vi "LVH5Rget_obj_type (DSet).vi"(6 "error in (no error)":errorcluster, 8 "HDF5 Object Reference":T2, 9 "HDF5 Location Ref":T3) -> (0 "error out":errorcluster, 2 "Object Type":T1 items=["H5O_TYPE_GROUP", "H5O_TYPE_DATASET", "H5O_NAMED_DATATYPE"], 3 "HDF5 Location Ref out":T3)   [LabVIEW 2017]
doc: "Retrieves the type of object that an object reference points to."
uses:
  <vilib>/UPVI/lvhdf5/library.llb/HDF5 Ref.ctl
  <vilib>/UPVI/lvhdf5/reference.llb/H5R Dataset Region Ref.ctl
  <vilib>/UPVI/lvhdf5/object.llb/H5O_type_t.ctl
  <vilib>/UPVI/lvhdf5/h5helper.dll
panel:
  # "LVHDF5 Toolkit\nCopyright (c) 2005-2013 by Jason D. Sommerville\nCopyright (c) 2014 by UPVI, LLC.\n\nThis use and distribution of this file is governed by the terms found in \nLICENSE.txt distributed with this toolkit and installed at\n <user.lib>\\_lvhdf5\\LICENSE.txt"
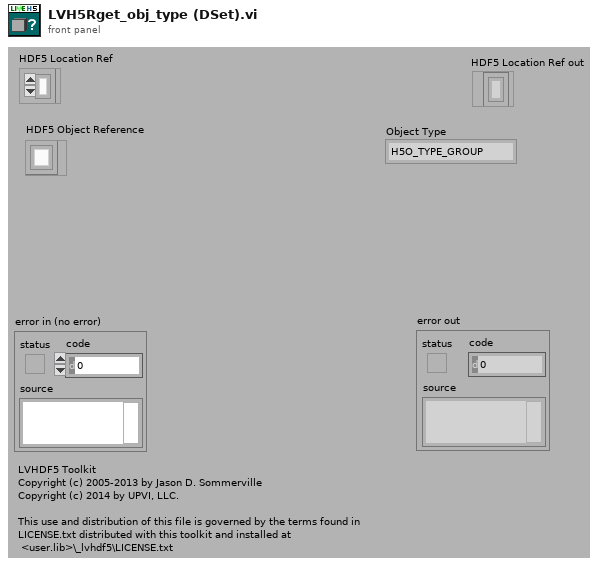
[diagram p1: front panel]
types:
  T1 = typedef "H5O_type_t.ctl" = i32
  T2 = typedef "H5R Dataset Region Ref.ctl" = refnum<k1>
  T3 = typedef "HDF5 Ref.ctl" = refnum<k1>
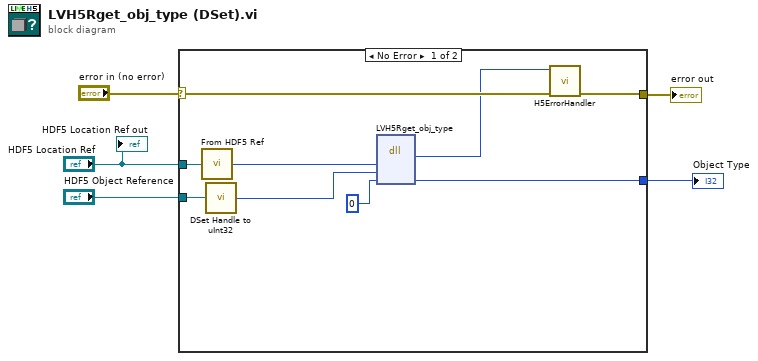
[diagram p0: block diagram]
diagram:
  n1 = case shown="No Error" "error in (no error)" {
    selector: "error in (no error)" -> [w14 w15]
    tunnel: [w13 w15] -> w4
    tunnel: "HDF5 Location Ref" -> [w12 _]
    tunnel: "HDF5 Object Reference" -> [w7 _]
    tunnel: [w8 _] -> w1
    frame No Error {
      n2 = call <vilib>:"From HDF5 Ref.vi"("HDF5 Ref"=w12) -> ("I32"=w11:i32)
      n3 = call <vilib>:"DSet Handle to uInt32.vi"("HDF5 Reference Type"=w7) -> ("Handle"=w6:u32)
      n4 = dll-call lib="C:/Program Files/National Instruments/LabVIEW 2017/vi.lib/UPVI/lvhdf5/h5helper.dll" fn="LVH5Rget_obj_type"("loc_id"=w11, "handle"=w6, "objtype"=u32 0) -> ("return type"=w10:i32, "objtype"=w8:u32)  [unwired: 5 in, 2 out]
      n5 = call <vilib>:"H5ErrorHandler.vi"("error in (no error)"=w14, "herr_t"=w10) -> ("error out"=w13:errorcluster)  [unwired: 3 in, 4 out]
    }
    frame Error {
    }
  }
  "error out" <- w4
  "Object Type" <- w1
  "HDF5 Location Ref out" <- "HDF5 Location Ref"
